vi "Convert Data to Items.vi"(8 "error in":errorcluster, 11 "OD Entry":T6={"index"=0, "sub-index"=0, "Level"=0, "ObjectType"=10, "DataType"=0, "ParameterName"="", "LowLimit"="", "HighLimit"="", "AccessType"=0, "DefaultValue"="", "PDOMapping"=FALSE, "SubNumber"=0, "ObjFlags"=0, "Category"=enum."Mandatory"} {"SubNumber" format="%x"; "AccessType" items=["", "ro", "wo", "rw", "const", "rwr", "rww"]; "DataType" items=[""=0, "BOOLEAN"=1, "INTEGER8"=2, "INTEGER16"=3, "INTEGER32"=4, "UNSIGNED8"=5, "UNSIGNED16"=6, "UNSIGNED32"=7, "REAL32"=8, "VISIBLE_STRING"=9, "OCTET_STRING"=10, "UNICODE_STRING"=11, "TIME_OF_DAY"=12, "TIME_DIFFERENCE"=13, "DOMAIN"=15, "INTEGER24"=16, "REAL64"=17, "INTEGER40"=18, "INTEGER48"=19, "INTEGER56"=20, "INTEGER64"=21, "UNSIGNED24"=22, "UNSIGNED40"=24, "UNSIGNED48"=25, "UNSIGNED56"=26, "UNSIGNED64"=27]; "ObjectType" items=[""=10, "NULL"=0, "DOMAIN"=2, "DEFTYPE"=5, "DEFSTRUCT"=6, "VAR"=7, "ARRAY"=8, "RECORD"=9]; "sub-index" format="%x"; "index" format="%x"}) -> (0 "error out":errorcluster, 3 "Item":T5)   [LabVIEW 2013]
uses:
  control/OD Entry.ctl
  control/Object Type.ctl
  control/Data Type.ctl
  control/Access Type.ctl
  control/OD Cateory.ctl
panel:
  out "Cateory":T1=enum.""
  out "0, 1":i16
  out "ObjFlags":u32
  out "AccessType":T2 items=["", "ro", "wo", "rw", "const", "rwr", "rww"]
  out "DataType":T3 items=[""=0, "BOOLEAN"=1, "INTEGER8"=2, "INTEGER16"=3, "INTEGER32"=4, "UNSIGNED8"=5, "UNSIGNED16"=6, "UNSIGNED32"=7, "REAL32"=8, "VISIBLE_STRING"=9, "OCTET_STRING"=10, "UNICODE_STRING"=11, "TIME_OF_DAY"=12, "TIME_DIFFERENCE"=13, "DOMAIN"=15, "INTEGER24"=16, "REAL64"=17, "INTEGER40"=18, "INTEGER48"=19, "INTEGER56"=20, "INTEGER64"=21, "UNSIGNED24"=22, "UNSIGNED40"=24, "UNSIGNED48"=25, "UNSIGNED56"=26, "UNSIGNED64"=27]
  out "ObjectType":T4=7 items=[""=10, "NULL"=0, "DOMAIN"=2, "DEFTYPE"=5, "DEFSTRUCT"=6, "VAR"=7, "ARRAY"=8, "RECORD"=9]
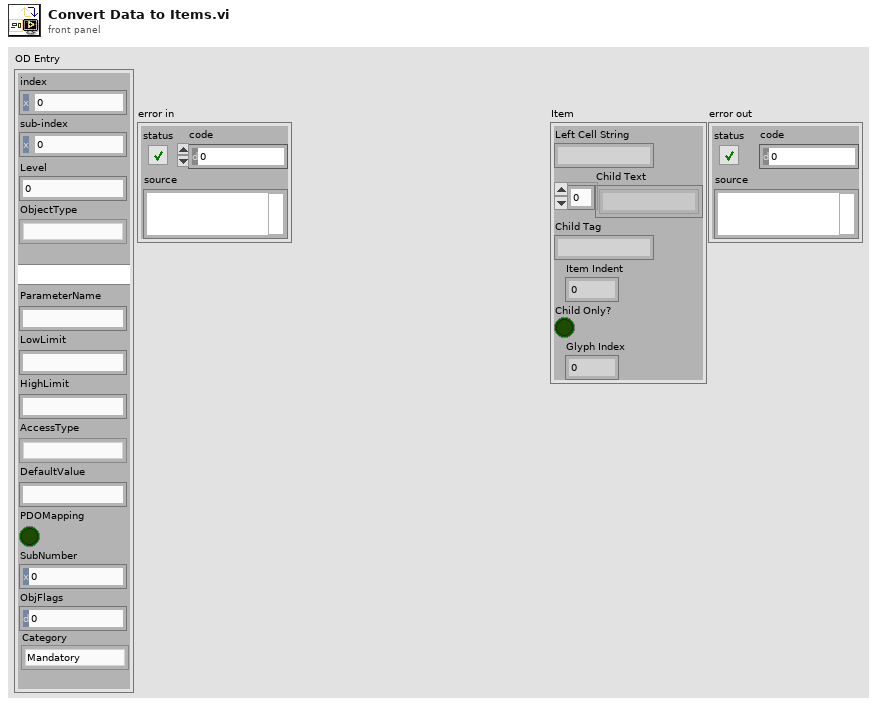
[diagram p1: front panel]
types:
  T1 = typedef "OD Cateory.ctl" = enum16{"Mandatory", "Optional", "Manufacturer", ""}
  T2 = typedef "Access Type.ctl" = u16
  T3 = typedef "Data Type.ctl" = u16
  T4 = typedef "Object Type.ctl" = u16
  T5 = cluster{"Left Cell String":string, "Child Text":string[], "Child Tag":string, "Item Indent":i32, "Child Only?":bool, "Glyph Index":i32}
  T6 = typedef "OD Entry.ctl" = cluster{"index":u16, "sub-index":u8, "Level":u8, "ObjectType":T4, "DataType":T3, "ParameterName":string, "LowLimit":string, "HighLimit":string, "AccessType":T2, "DefaultValue":string, "PDOMapping":bool, "SubNumber":u8, "ObjFlags":u32, "Category":T1}
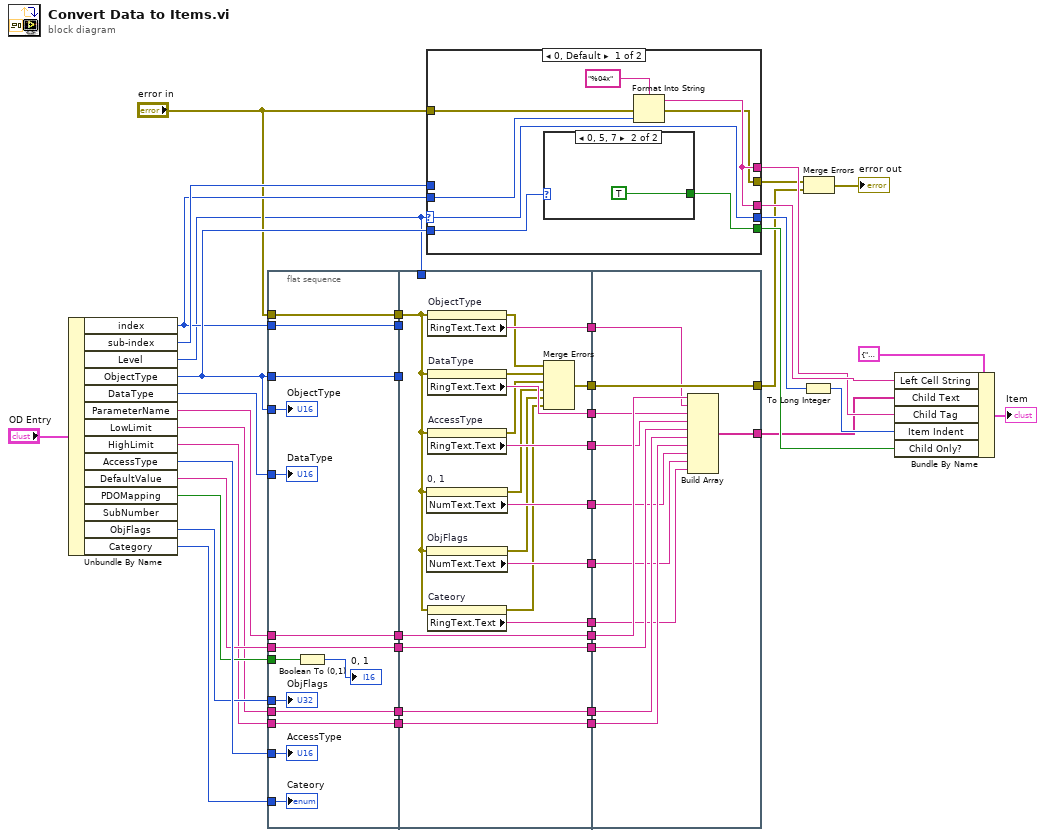
[diagram p0: block diagram]
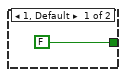
[diagram p2: hidden frame]
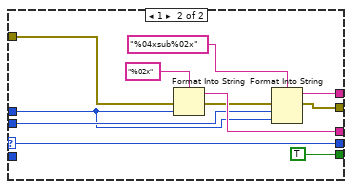
[diagram p3: hidden frame]
diagram:
  n1 = Unbundle By Name("OD Entry") -> ("index"=w5:u16, "sub-index"=w36:u8, "Level"=w3:u8, "ObjectType"=w21:T4, "DataType"=w34:T3, "ParameterName"=w27:string, "LowLimit"=w28:string, "HighLimit"=w29:string, "AccessType"=w33:T2, "DefaultValue"=w31:string, "PDOMapping"=w30:bool, "ObjFlags"=w32:u32, "Category"=w2:T1)  [unwired: 1 out]
  n2 = flat-sequence {
    tunnel: w21 -> [w58]
    tunnel: w34 -> [w57]
    tunnel: w33 -> [w56]
    tunnel: w32 -> [w55]
    tunnel: w31 -> [w49]
    tunnel: w30 -> [w54]
    tunnel: w29 -> [w50]
    tunnel: w28 -> [w51]
    tunnel: w27 -> [w52]
    tunnel: [w52] -> w26
    tunnel: [w51] -> w25
    tunnel: [w50] -> w24
    tunnel: [w49] -> w23
    tunnel: w21 -> [w48]
    tunnel: [w48] -> w22
    tunnel: "error in" -> [w47]
    tunnel: [w47] -> w20
    tunnel: [w46] -> w6
    tunnel: w5 -> [w46]
    tunnel: w2 -> [w45]
    tunnel: w26 -> [w76]
    tunnel: w25 -> [w75]
    tunnel: w24 -> [w74]
    tunnel: w23 -> [w73]
    tunnel: w22 -> [_]
    tunnel: w20 -> [w61]
    tunnel: [w76] -> w18
    tunnel: [w75] -> w17
    tunnel: [w74] -> w16
    tunnel: [w73] -> w15
    tunnel: [w72] -> w14
    tunnel: [w71] -> w13
    tunnel: [w70] -> w12
    tunnel: [w69] -> w11
    tunnel: [w63] -> w10
    tunnel: [w62] -> w9
    tunnel: w6 -> [_]
    tunnel: w3 -> [_]
    tunnel: [w59] -> w1
    tunnel: [w88] -> w8
    tunnel: w18 -> [w87]
    tunnel: w17 -> [w82]
    tunnel: w16 -> [w81]
    tunnel: w15 -> [w83]
    tunnel: w14 -> [w86]
    tunnel: w13 -> [w85]
    tunnel: w12 -> [w84]
    tunnel: w11 -> [w80]
    tunnel: w10 -> [w79]
    tunnel: w9 -> [w88]
    tunnel: [w78] -> w7
    tunnel: w1 -> [w77]
    frame #0 {
      n3 = Boolean To (0,1)(Boolean=w54) -> (0, 1=→"0, 1":i16)
      "ObjectType" <- w58
      "DataType" <- w57
      "AccessType" <- w56
      "ObjFlags" <- w55
      "Cateory" <- w45
    }
    frame #1 {
      n4 = property on="0, 1" class="DigNum (strict)"(error in=w61) -> (error out=w65:errorcluster, "NumText.Text"=w69:string)  [unwired: 1 in, 1 out]
      n5 = property on="ObjFlags" class="DigNum (strict)"(error in=w61) -> (error out=w64:errorcluster, "NumText.Text"=w63:string)  [unwired: 1 in, 1 out]
      n6 = property on="ObjectType" class="Ring (strict)"(error in=w61) -> (error out=w68:errorcluster, "RingText.Text"=w72:string)  [unwired: 1 in, 1 out]
      n7 = property on="DataType" class="Ring (strict)"(error in=w61) -> (error out=w67:errorcluster, "RingText.Text"=w71:string)  [unwired: 1 in, 1 out]
      n8 = property on="AccessType" class="Ring (strict)"(error in=w61) -> (error out=w66:errorcluster, "RingText.Text"=w70:string)  [unwired: 1 in, 1 out]
      n9 = property on="Cateory" class="Enum (strict)"(error in=w61) -> (error out=w60:errorcluster, "RingText.Text"=w59:string)  [unwired: 1 in, 1 out]
      n10 = Merge Errors(w68, w67, w66, w65, w64, w60) -> (w62:errorcluster)
    }
    frame #2 {
      n11 = Build Array(w87, w86, w85, w84, w83, w82, w81, w80, w79, w77) -> (w78:string[])
    }
  }
  n12 = case shown="0, Default" w3 {
    selector: w3 -> [w93 w102]
    tunnel: w5 -> [w95 w105]
    tunnel: [w94 w108] -> w41
    tunnel: [w94 w103] -> w40
    tunnel: [w89 TRUE] -> w39
    tunnel: [w93 w102] -> w38
    tunnel: "error in" -> [w92 w107]
    tunnel: [w91 w99] -> w37
    tunnel: w36 -> [_ w104]
    tunnel: w21 -> [w90 _]
    frame 0, Default {
      n13 = case shown="0, 5, 7" w90 {
        tunnel: [FALSE TRUE] -> w89
        frame 1, Default {
        }
        frame 0, 5, 7 {
        }
      }
      n14 = Format Into String(format string="%04x", error in=w92, w95) -> (resulting string=w94:string, error out=w91:errorcluster)  [unwired: 1 in]
    }
    frame 1 {
      n15 = Format Into String(format string="%02x", error in=w107, w104) -> (resulting string=w108:string, error out=w100:errorcluster)  [unwired: 1 in]
      n16 = Format Into String(format string="%04xsub%02x", error in=w100, w105, w104) -> (resulting string=w103:string, error out=w99:errorcluster)  [unwired: 1 in]
    }
  }
  n17 = To Long Integer(number=w38) -> (32bit integer=w35:i32)
  n18 = Merge Errors(w37, w8) -> (→"error out":errorcluster)
  n19 = Bundle By Name(cluster=T5 {"Left Cell String"="", "Child Text"=[], "Child Tag"="", "Item Indent"=0, "Child Only?"=FALSE, "Glyph Index"=0} ("Item 2"), "Left Cell String"=w41, "Child Text"=w7, "Child Tag"=w40, "Item Indent"=w35, "Child Only?"=w39) -> (→"Item":T5)
